vi "Obtain Request Events.vi"(8 "error in (no error)":errorcluster, 10 "Create New? (F)":bool) -> (0 "error out":errorcluster, 2 "Analysis Request Events":T1)   [LabVIEW 2019, in "Analysis.lvlib"]
doc: "This VI Obtains/Creates the Requests events that will be used for other modules to communicate with the module that owns this VI. These Requests events will be accessed only via Public API methods for this module.\n\n<b>NOTE</b>: The contents of this VI are automatically generated and modified by the <b>Tools > Delacor > DQMH</b> utilities. Consider using those utilities instead of making your own modifications to this VI.\n_____\nBased on Delacor QMH Project Template 4.0.0.47.\n_____\nBased on DQMH Project Template 6.1.0.94."
uses:
  Analysis.lvlib
  Request Events--cluster.ctl
  Stop Argument--cluster.ctl
  Show Panel Argument--cluster.ctl
  Hide Panel Argument--cluster.ctl
  Get Module Execution Status Argument--cluster.ctl
  Show Diagram Argument--cluster.ctl
  Wakeup Helper Loop Argument--cluster.ctl
  Change Settings Argument--cluster.ctl
  Main UI Shared/Signal Type--enum.ctl
  Main UI Shared/Calibration Values--cluster.ctl
  Update analysis parameters Argument--cluster.ctl
  Main UI Shared/Decimation input --cluster.ctl
  Update analysis parameters (Reply Payload)--cluster.ctl
  Update Savitzky parameters Argument--cluster.ctl
  Update decimation Argument--cluster.ctl
  Update contact parameters Argument--cluster.ctl
  Update Tau delay (ms) Argument--cluster.ctl
  Open Fcurve object Argument--cluster.ctl
  Neo-Laura-LVOOP/SignalViewer/TDMS_DataHandler_class/Fcurve Meta data.ctl
  Open Fcurve object (Reply Payload)--cluster.ctl
  Neo-Laura-LVOOP/Class Library/Fcurve_class/Metadata.ctl
  Apply Savitzky Golay Filter Argument--cluster.ctl
  Apply Savitzky Golay Filter (Reply Payload)--cluster.ctl
  Apply decimation Argument--cluster.ctl
  Apply decimation (Reply Payload)--cluster.ctl
  Main UI Shared/MAIN UI Shared.lvlib
  Neo-Laura-LVOOP/SignalViewer/TDMS_DataHandler_class/TDMS_DataHandler.lvclass
  Neo-Laura-LVOOP/Class Library/Fcurve_class/Fcurve.lvclass
panel:
  # "NOTE: The contents of this VI are automatically generated and modified by the Tools > Delacor > DQMH utilities. Consider using those utilities instead of making your own modifications to this VI."
  # "Contact"
  # "Contact"
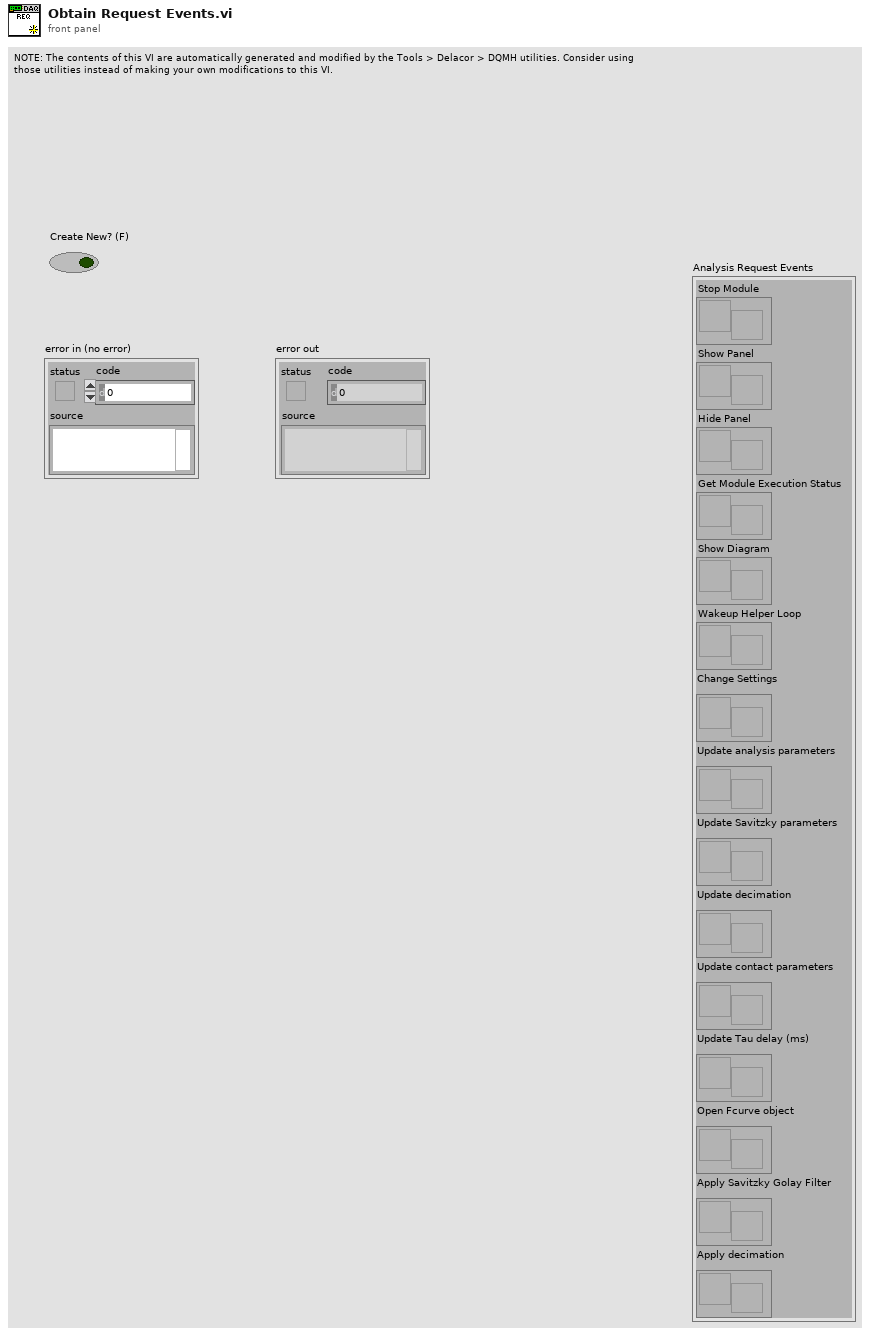
[diagram p1: front panel]
types:
  T1 = typedef "Analysis.lvlib/Request Events--cluster.ctl" = cluster{"Stop Module":refnum<user-event>, "Show Panel":refnum<user-event>, "Hide Panel":refnum<user-event>, "Get Module Execution Status":refnum<user-event>, "Show Diagram":refnum<user-event>, "Wakeup Helper Loop":refnum<user-event>, "Change Settings":refnum<user-event>, "Update analysis parameters":refnum<user-event>, "Update Savitzky parameters":refnum<user-event>, "Update decimation":refnum<user-event>, "Update contact parameters":refnum<user-event>, "Update Tau delay (ms)":refnum<user-event>, "Open Fcurve object":refnum<user-event>, "Apply Savitzky Golay Filter":refnum<user-event>, "Apply decimation":refnum<user-event>}
  T2 = typedef "Analysis.lvlib/Apply decimation Argument--cluster.ctl" = cluster{"Ch Datum":waveform(dbl)[], "Wait Notifier":refnum<notifier>, "wait for reply":bool}
  T3 = typedef "Analysis.lvlib/Apply Savitzky Golay Filter Argument--cluster.ctl" = cluster{"Ch Datum":waveform(dbl)[], "Wait Notifier":refnum<notifier>, "wait for reply":bool}
  T4 = typedef "Analysis.lvlib/Open Fcurve object Argument--cluster.ctl" = cluster{"Group metadata":T5, "Channel name(s)":string[], "Channel datum out":waveform(dbl)[], "Wait Notifier":refnum<notifier>, "wait for reply":bool}
  T5 = typedef "TDMS_DataHandler.lvclass/Fcurve Meta data.ctl" = cluster{"property names":string[], "property values":variant[]}
  T6 = typedef "Analysis.lvlib/Update Tau delay (ms) Argument--cluster.ctl" = cluster{"Tau Delay (ms)":dbl}
  T7 = typedef "Analysis.lvlib/Update contact parameters Argument--cluster.ctl" = cluster{"Contact":cluster{"Contact stat?":bool, "Contact Spread of dev":dbl}}
  T8 = typedef "Analysis.lvlib/Update decimation Argument--cluster.ctl" = cluster{"Decimation":T9}
  T9 = typedef "MAIN UI Shared.lvlib/Decimation input --cluster.ctl" = cluster{"App":cluster{"Dec":i32, "apply":bool}, "Con":cluster{"Dec":i32, "apply":bool}, "Ret":cluster{"Dec":i32, "apply":bool}}
  T10 = typedef "Analysis.lvlib/Update Savitzky parameters Argument--cluster.ctl" = cluster{"Savitzksky-Golay":cluster{"Sidepoints (M)":dbl, "Filter Order":i32}}
  T11 = typedef "Analysis.lvlib/Update analysis parameters Argument--cluster.ctl" = cluster{"Contact":cluster{"Contact stat?":bool, "Contact Spread of dev":dbl}, "Decimation":T9, "Savitzksky-Golay":cluster{"Sidepoints (M)":dbl, "Filter Order":i32}, "Wait Notifier":refnum<notifier>, "wait for reply":bool}
  T12 = typedef "Analysis.lvlib/Change Settings Argument--cluster.ctl" = cluster{"Signal Type":T13, "Calibration Array":T14[]}
  T13 = typedef "MAIN UI Shared.lvlib/Signal Type--enum.ctl" = enum16{"Sine Wave", "Square with Noise"}
  T14 = typedef "MAIN UI Shared.lvlib/Calibration Values--cluster.ctl" = cluster{"Slope":dbl, "Offset":dbl}
  T15 = typedef "Analysis.lvlib/Wakeup Helper Loop Argument--cluster.ctl" = cluster{"HW ID":string}
  T16 = typedef "Analysis.lvlib/Hide Panel Argument--cluster.ctl" = cluster{"Hide Panel?":bool}
  T17 = typedef "Analysis.lvlib/Show Panel Argument--cluster.ctl" = cluster{"Show Panel?":bool}
  T18 = typedef "Analysis.lvlib/Show Diagram Argument--cluster.ctl" = cluster{"Debug?":bool}
  T19 = typedef "Analysis.lvlib/Get Module Execution Status Argument--cluster.ctl" = cluster{"Running?":bool}
  T20 = typedef "Analysis.lvlib/Stop Argument--cluster.ctl" = cluster{"Origin":string, "Exit via Stop Module Req?":bool, "Wait for Module to stop?":bool}
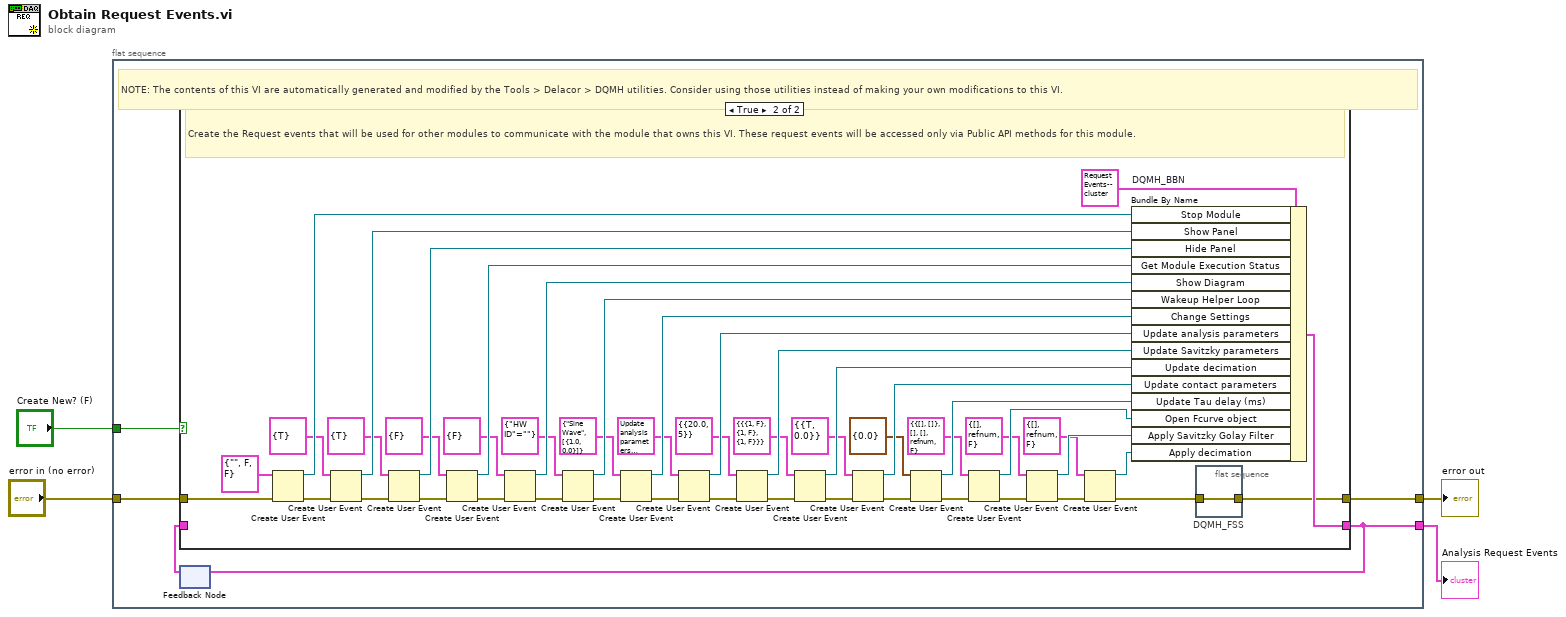
[diagram p0: block diagram]
diagram:
  n1 = flat-sequence {
    tunnel: [w9] -> w4
    tunnel: "error in (no error)" -> [w8]
    tunnel: [w6] -> w2
    tunnel: "Create New? (F)" -> [w5]
    frame #0 {
      # "NOTE: The contents of this VI are automatically generated and modified by the Tools > Delacor > DQMH utilities. Consider using those utilities instead of making your own modifications to this VI."
      n2 = feedback #1() -> (w7:T1)  [unwired: 1 in]
      n3 = case shown="True" w5 {
        tunnel: [w10 w50] -> w9
        tunnel: w8 -> [w10 w60]
        tunnel: [w11 w57] -> w6
        tunnel: w7 -> [w11 _]
        frame False {
          # "Obtain the Request events that were created in a previous call to this VI."
        }
        frame True {
          # "Create the Request events that will be used for other modules to communicate with the module that owns this VI. These request events will be accessed only via Public API methods for this module."
          n4 = Create User Event(user event datatype=T20 {"Origin"="", "Exit via Stop Module Req?"=FALSE, "Wait for Module to stop?"=FALSE} ("Stop Argument"), error in=w60) -> (user event=w58:refnum<user-event>, error out=w55:errorcluster)
          n5 = Create User Event(user event datatype=T17 {"Show Panel?"=TRUE} ("Show Panel Argument"), error in=w55) -> (user event=w54:refnum<user-event>, error out=w53:errorcluster)
          n6 = Create User Event(user event datatype=T16 {"Hide Panel?"=TRUE} ("Hide Panel Argument"), error in=w53) -> (user event=w52:refnum<user-event>, error out=w51:errorcluster)
          n7 = Create User Event(user event datatype=T19 {"Running?"=FALSE} ("Get Module Execution Status Argument"), error in=w51) -> (user event=w48:refnum<user-event>, error out=w49:errorcluster)
          n8 = Create User Event(user event datatype=T18 {"Debug?"=FALSE} ("Show Diagram Argument"), error in=w49) -> (user event=w45:refnum<user-event>, error out=w46:errorcluster)
          n9 = Create User Event(user event datatype=T15 {"HW ID"=""} ("Wakeup Message Pump Argument"), error in=w46) -> (user event=w40:refnum<user-event>, error out=w41:errorcluster)
          n10 = Create User Event(user event datatype=T12 {"Signal Type"=enum."Sine Wave", "Calibration Array"=[{"Slope"=1.0, "Offset"=0.0}]} ("Change Settings Argument"), error in=w41) -> (user event=w37:refnum<user-event>, error out=w38:errorcluster)
          n11 = Create User Event(user event datatype=T11 {"Contact"={"Contact stat?"=TRUE, "Contact Spread of dev"=0.0}, "Decimation"={"App"={"Dec"=1, "apply"=FALSE}, "Con"={"Dec"=1, "apply"=FALSE}, "Ret"={"Dec"=1, "apply"=FALSE}}, "Savitzksky-Golay"={"Sidepoints (M)"=20.0, "Filter Order"=5}, "Wait Notifier"=refnum, "wait for reply"=FALSE} ("Update analysis parameters Argument"), error in=w38) -> (user event=w34:refnum<user-event>, error out=w35:errorcluster)
          n12 = Create User Event(user event datatype=T10 {"Savitzksky-Golay"={"Sidepoints (M)"=20.0, "Filter Order"=5}} ("Update Savitzky parameters Argument"), error in=w35) -> (user event=w31:refnum<user-event>, error out=w32:errorcluster)
          n13 = Create User Event(user event datatype=T8 {"Decimation"={"App"={"Dec"=1, "apply"=FALSE}, "Con"={"Dec"=1, "apply"=FALSE}, "Ret"={"Dec"=1, "apply"=FALSE}}} ("Update decimation Argument"), error in=w32) -> (user event=w28:refnum<user-event>, error out=w29:errorcluster)
          n14 = Create User Event(user event datatype=T7 {"Contact"={"Contact stat?"=TRUE, "Contact Spread of dev"=0.0}} ("Update contact parameters Argument"), error in=w29) -> (user event=w25:refnum<user-event>, error out=w26:errorcluster)
          n15 = Create User Event(user event datatype=T6 {"Tau Delay (ms)"=0.0} ("Update Tau delay (ms) Argument"), error in=w26) -> (user event=w22:refnum<user-event>, error out=w23:errorcluster)
          n16 = Create User Event(user event datatype=T4 {"Group metadata"={"property names"=[], "property values"=[]}, "Channel name(s)"=[], "Channel datum out"=[], "Wait Notifier"=refnum, "wait for reply"=FALSE} ("Open Fcurve object Argument"), error in=w23) -> (user event=w19:refnum<user-event>, error out=w20:errorcluster)
          n17 = Create User Event(user event datatype=T3 {"Ch Datum"=[], "Wait Notifier"=refnum, "wait for reply"=FALSE} ("Apply Savitzky Golay Filter Argument"), error in=w20) -> (user event=w16:refnum<user-event>, error out=w17:errorcluster)
          n18 = Create User Event(user event datatype=T2 {"Ch Datum"=[], "Wait Notifier"=refnum, "wait for reply"=FALSE} ("Apply decimation Argument"), error in=w17) -> (user event=w13:refnum<user-event>, error out=w14:errorcluster)
          n19 = Bundle By Name "DQMH_BBN"(cluster=T1 {"Stop Module"=refnum, "Show Panel"=refnum, "Hide Panel"=refnum, "Get Module Execution Status"=refnum, "Show Diagram"=refnum, "Wakeup Helper Loop"=refnum, "Change Settings"=refnum, "Update analysis parameters"=refnum, "Update Savitzky parameters"=refnum, "Update decimation"=refnum, "Update contact parameters"=refnum, "Update Tau delay (ms)"=refnum, "Open Fcurve object"=refnum, "Apply Savitzky Golay Filter"=refnum, "Apply decimation"=refnum} ("output cluster"), "Stop Module"=w58, "Show Panel"=w54, "Hide Panel"=w52, "Get Module Execution Status"=w48, "Show Diagram"=w45, "Wakeup Helper Loop"=w40, "Change Settings"=w37, "Update analysis parameters"=w34, "Update Savitzky parameters"=w31, "Update decimation"=w28, "Update contact parameters"=w25, "Update Tau delay (ms)"=w22, "Open Fcurve object"=w19, "Apply Savitzky Golay Filter"=w16, "Apply decimation"=w13) -> (w57:T1)
          n20 = flat-sequence "DQMH_FSS" {
            tunnel: w14 -> [w61]
            tunnel: [w61] -> w50
            frame #0 {
            }
          }
        }
      }
      n21 = feedback-in #1(w6) -> ()
    }
  }
  "Analysis Request Events" <- w2
  "error out" <- w4
